vi "Open Audio File Read.vi"(8 "error in (no error)":errorcluster, 11 "Path":path) -> (0 "error out":errorcluster, 3 "Audio File Refnum":refnum<file>)   [LabVIEW 2020, in "G-Audio.lvlib"]
doc: "Opens an audio file and initializes the relevant decoder. If <b>codec</b> isn't specified, file extension determines the codec type.\n\nSupported codecs: flac, mp3, vorbis (ogg), and wav."
uses:
  G-Audio.lvlib
  Private/Get File Extension (Reentrant).vi
  <vilib>/Utility/error.llb/Error Cluster From Error Code.vi
  <vilib>/Utility/file.llb/Application Directory.vi
  lib/g_audio_x86.dll
  lib/g_audio_x64.dll
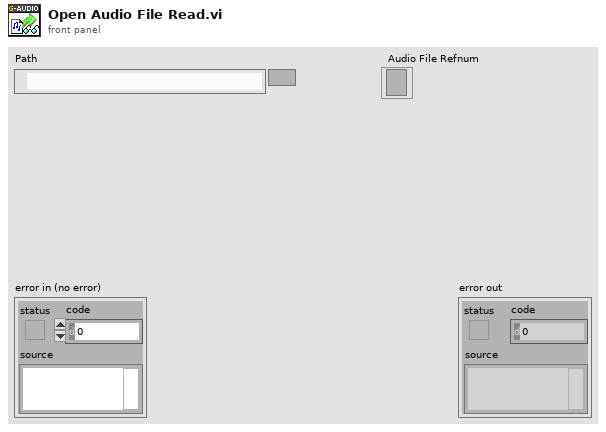
[diagram p1: front panel]
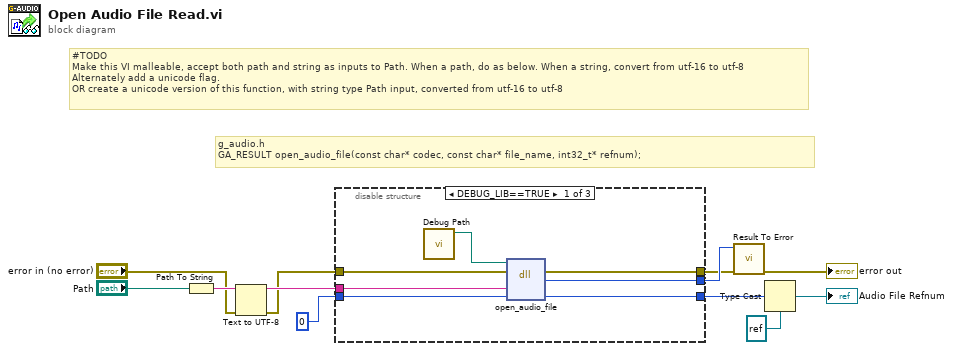
[diagram p0: block diagram]
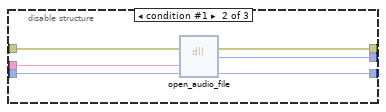
[diagram p2: hidden frame]
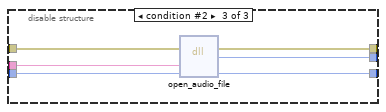
[diagram p3: hidden frame]
diagram:
  # "#TODO\nMake this VI malleable, accept both path and string as inputs to Path. When a path, do as below. When a string, convert from utf-16 to utf-8\nAlternately add a unicode flag.\nOR create a unicode version of this function, with string type Path input, converted from utf-16 to utf-8"
  # "g_audio.h\nGA_RESULT open_audio_file(const char* codec, const char* file_name, int32_t* refnum);"
  n1 = Path To String(path="Path") -> (string=w5:string)
  n2 = Text to UTF-8(8:"error in (no error)", 11:w5) -> (0:w3:errorcluster, 3:w4:string)  [unwired: 1 in]
  n3 = disable-structure shown="DEBUG_LIB==TRUE" {
    disable-tunnel: w3 -> [w19 w25 w31]
    disable-tunnel: w4 -> [w17 w23 w29]
    disable-tunnel: [w18 w24 w30] -> w7
    disable-tunnel: 0 ("num_samples") -> [w16 w22 w28]
    disable-tunnel: [w15 w21 w27] -> w10
    disable-tunnel: [w14 w20 w26] -> w8
    frame condition #0 (active) {
      n4 = call "Debug Path.vi"() -> ("Debug Path"=w13:path)  [unwired: 11 in]
      n5 = dll-call lib="?" fn="open_audio_file"(path in=w13, error in=w19, "file_name"=w17, "refnum"=w16) -> (error out=w18:errorcluster, "result"=w14:i32, "refnum"=w15:i32)  [unwired: 2 in, 1 out]
    }
    frame condition #1 {
      n6 = dll-call lib="C:/github/dataflowg/g-audio/src/LabVIEW/G-Audio/lib/g_audio_x86.*" fn="open_audio_file"(error in=w25, "file_name"=w23, "refnum"=w22) -> (error out=w24:errorcluster, "result"=w20:i32, "refnum"=w21:i32)  [unwired: 3 in, 1 out]
    }
    frame condition #2 {
      n7 = dll-call lib="C:/github/dataflowg/g-audio/src/LabVIEW/G-Audio/lib/g_audio_x64.*" fn="open_audio_file"(error in=w31, "file_name"=w29, "refnum"=w28) -> (error out=w30:errorcluster, "result"=w26:i32, "refnum"=w27:i32)  [unwired: 3 in, 1 out]
    }
  }
  n8 = call "Result To Error.vi"("error in (no error)"=w7, "Result Code"=w8) -> ("error out"=→"error out":errorcluster)  [unwired: 9 in]
  n9 = Type Cast(type=refnum<file> refnum ("Audio File Refnum"), x=w10) -> (*(type *) &x=→"Audio File Refnum":refnum<file>)
